vi "SuperSimple.vi"() -> ()   [LabVIEW 2020]
panel:
  out "return value 2":bool
  in  "stop":bool
  out "return value":bool
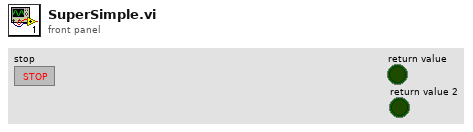
[diagram p1: front panel]
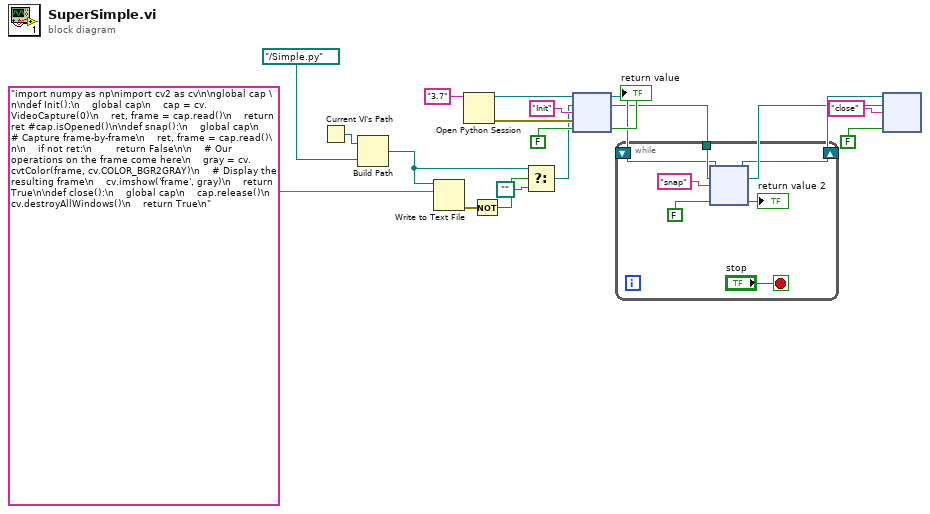
[diagram p0: block diagram]
diagram:
  n1 = Current VI's Path() -> (path=w10:path)
  n2 = Build Path(base path=w10, name or relative path=path "../Simple.py") -> (appended path=w17:path)
  n3 = Write to Text File(file (use dialog)=w17, text="import numpy as np\nimport cv2 as cv\n\nglobal cap \n\ndef Init():\n    global cap\n    cap = cv.VideoCapture(0)\n    ret, frame = cap.read()\n    return  ret #cap.isOpened()\n\ndef snap():\n    global cap\n    # Capture frame-by-frame\n    ret, frame = cap.read()\n\n    if not ret:\n        return False\n\n    # Our operations on the frame come here\n    gray = cv.cvtColor(frame, cv.COLOR_BGR2GRAY)\n    # Display the resulting frame\n    cv.imshow('frame', gray)\n    return True\n\ndef close():\n    global cap\n    cap.release()\n    cv.destroyAllWindows()\n    return True\n") -> (error out=w14:errorcluster)  [unwired: 2 in, 2 out]
  n4 = Open Python Session(python version="3.7" ("Python version")) -> (session out=w18:refnum<k35>, error out=w13:errorcluster)  [unwired: 2 in]
  n5 = Not(x=w14) -> (.not. x?=w15:bool)
  n6 = Select(t=w17, s=w15, f=path "") -> (s? t:f=w1:path)
  n7 = node(w18, w1, "Init" ("function name"), w13, FALSE) -> (w3:refnum<k35>, →"return value":bool)  [unwired: 3 out]
  n8 = while {
    tunnel: w1 -> [w21]
    shift-right: [w22] -> w2
    shift-left: w3 -> [w23]
    stop <- "stop" stop-if-true
    n9 = node(w23, w21, "snap" ("function name"), FALSE) -> (w22:refnum<k35>, →"return value 2":bool)  [unwired: 1 in, 3 out]
  }
  n10 = node(w2, w1, "close" ("function name"), FALSE) -> ()  [unwired: 2 in, 4 out]
